vi "subDAQ_GenWaveform.vi"(7 "Waveform port selection":T2={"Dev2 DO lines"=["Dev2/port0/line3", "Dev2/port0/line5"], "Dev2 AO lines"=["Dev2/ao3", "Dev2/ao5"], "Patch AO line"="Dev1/ao0", "Dev1 AI lines"=["Dev1/ai0", "Dev1/ai8"], "Dev1 timing DO"="Dev1/port0/line1", "Camera timing DI"="Dev1/port0/line0", "Dev1 trigger source"="/Dev1/PFI0", "Dev2 trigger source"="/Dev2/PFI0"}, 8 "error in (no error)":errorcluster, 11 "Waveform info":T3={"Waveform folder"=path "C:/Users/ZouOptics/Desktop/MATLAB codes/ephys waveforms_new/Voltage triangle -100 to +50_(Baseline -30)", "Exposure time (ms)"=10.0} {"Exposure time (ms)" format="%0.5f"}) -> (0 "error out":errorcluster, 1 "Dev1 AO waveform":waveform(dbl)(graph)={"t0"=timestamp(0 s since 1904-01-01), "dt"=inf, "Y"=[]}, 2 "Lasers AO waveform":waveform(dbl)[](graph)=[{"t0"=timestamp(0 s since 1904-01-01), "dt"=inf, "Y"=[]}, {"t0"=timestamp(0 s since 1904-01-01), "dt"=inf, "Y"=[]}], 3 "Lasers DO waveform":digitalwaveform[](graph)=[{"t0"=timestamp(0 s since 1904-01-01), "dt"=inf, "Y"={"transitions"=[], "data"=[]}}, {"t0"=timestamp(0 s since 1904-01-01), "dt"=inf, "Y"={"transitions"=[], "data"=[]}}], 4 "Acquisition params":T1={"Sampling rate (Hz)"=0.0, "dt (sec)"=0.0, "total time (sec)"=0.0, "# samples"=0, "Exposure time (ms)"=1000.0, "# frames"=0} {"Exposure time (ms)" format="%0.5f"; "Sampling rate (Hz)" format="%#.3f"})   [LabVIEW 2015]
uses:
  <vilib>/Utility/file.llb/Read Delimited Spreadsheet (DBL).vi
  <vilib>/Waveform/DWDTOps.llb/DWDT Analog to Digital.vi
panel:
  in  "waveform info name":string="waveform info.txt"
  in  "waveform data name":string="waveform data.txt"
  # "Read from text file and convert columns into waveforms"
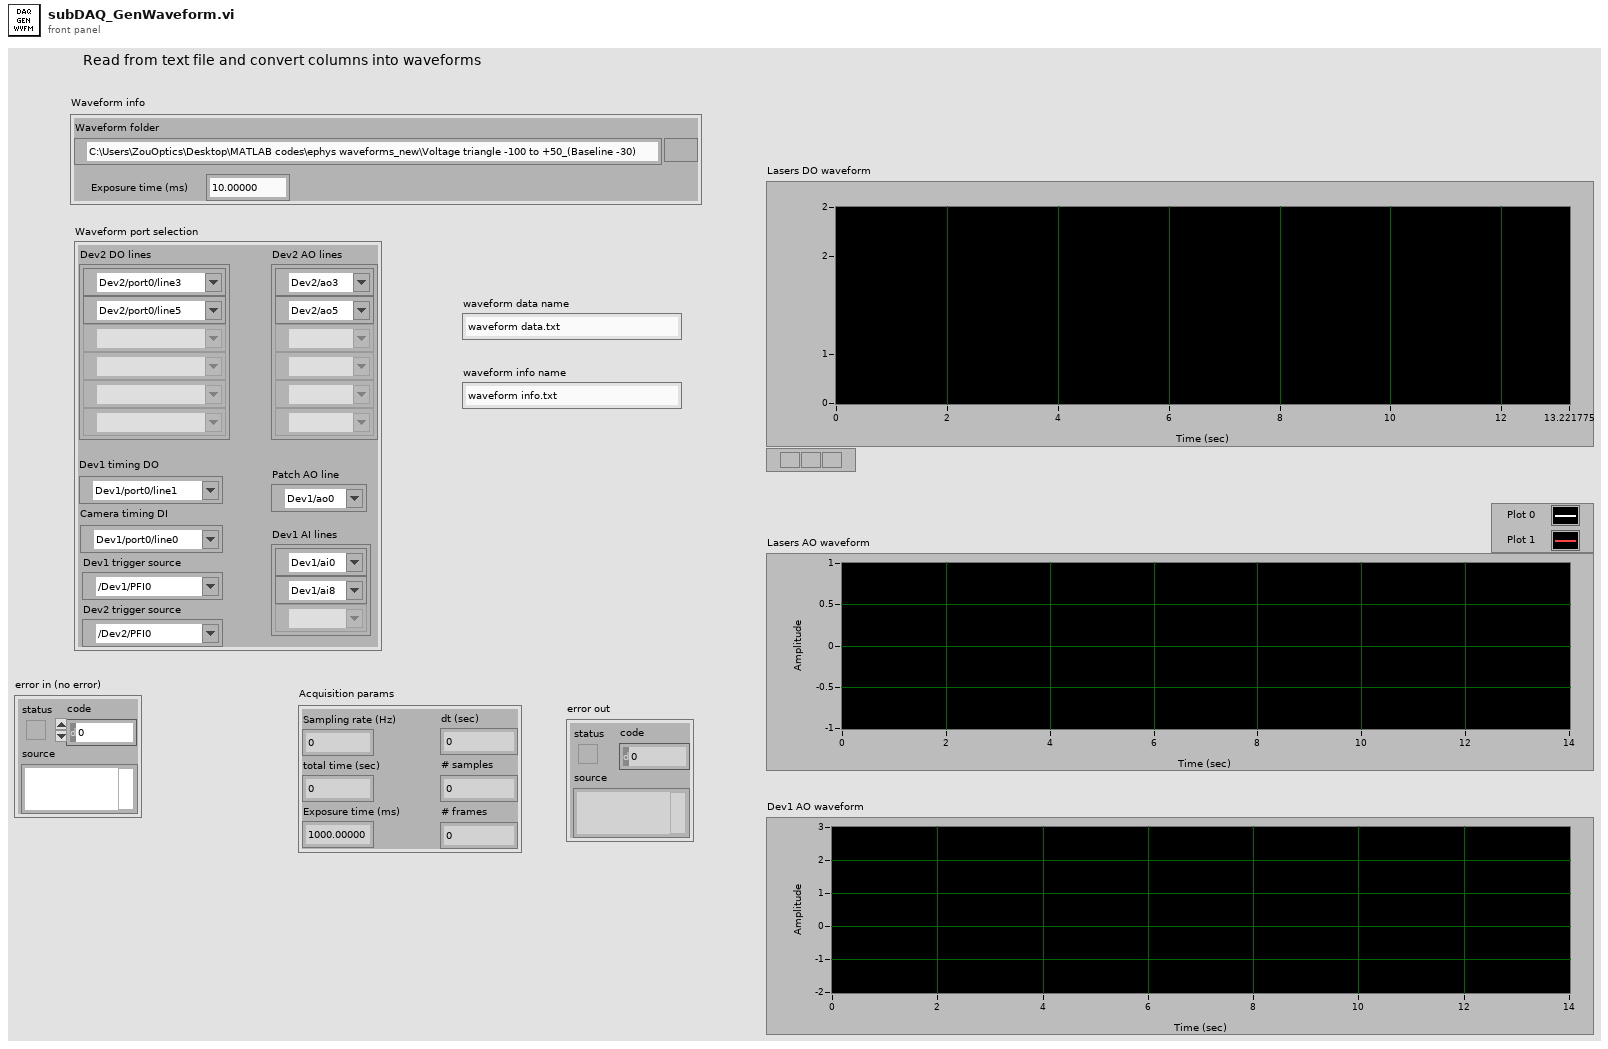
[diagram p1: front panel]
types:
  T1 = cluster{"Sampling rate (Hz)":dbl, "dt (sec)":dbl, "total time (sec)":dbl, "# samples":i32, "Exposure time (ms)":dbl, "# frames":i32}
  T2 = cluster{"Dev2 DO lines":tag[], "Dev2 AO lines":tag[], "Patch AO line":tag, "Dev1 AI lines":tag[], "Dev1 timing DO":tag, "Camera timing DI":tag, "Dev1 trigger source":tag, "Dev2 trigger source":tag}
  T3 = cluster{"Waveform folder":path, "Exposure time (ms)":dbl}
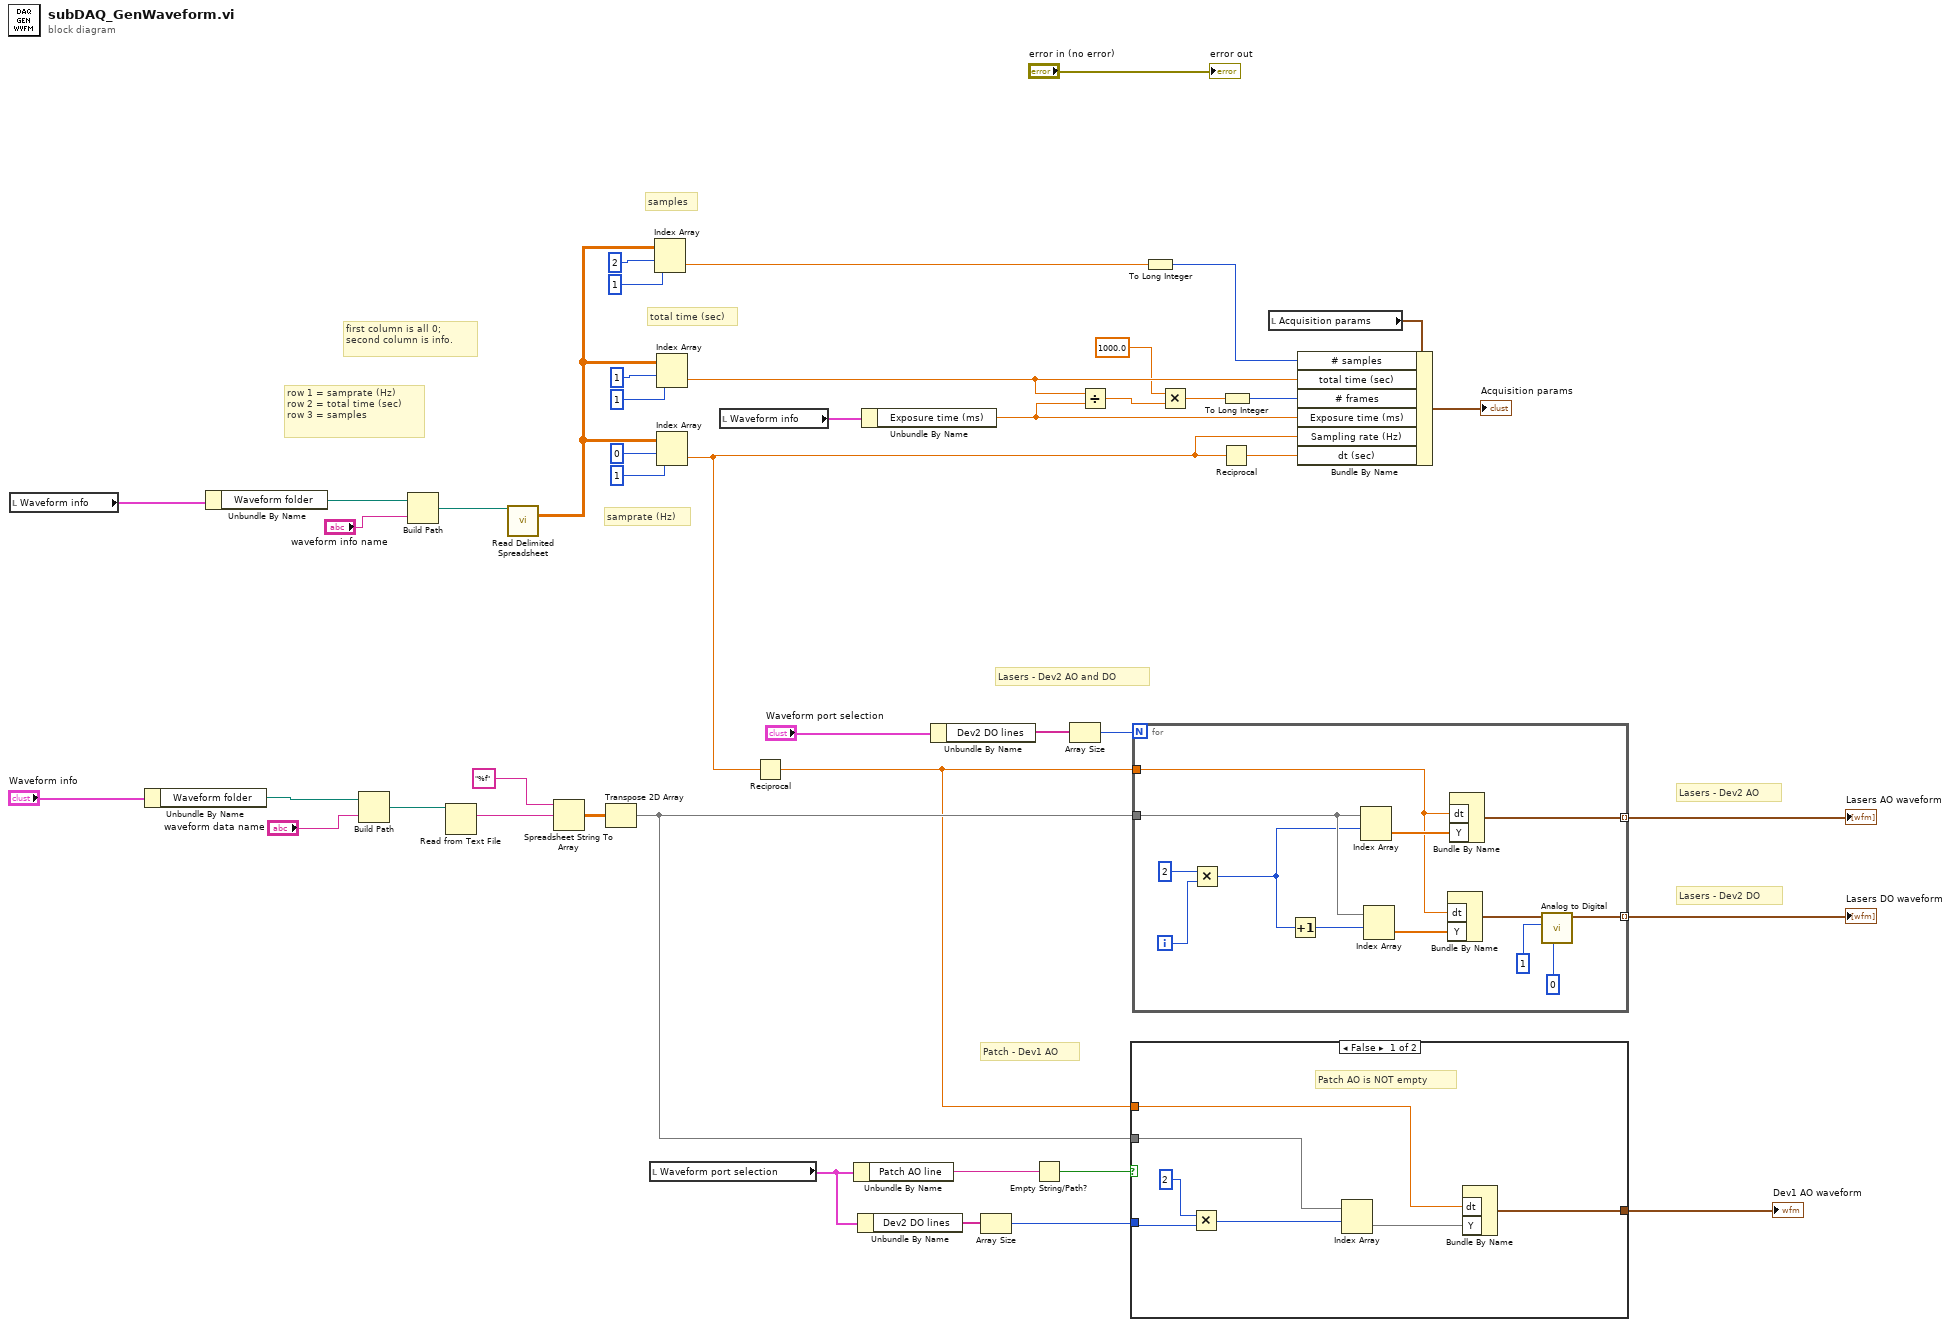
[diagram p0: block diagram]
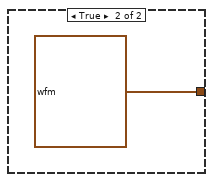
[diagram p2: hidden frame]
diagram:
  # "total time (sec)"
  # "samprate (Hz)"
  # "samples"
  # "Lasers - Dev2 AO and DO"
  # "first column is all 0;\nsecond column is info."
  # "row 1 = samprate (Hz)\nrow 2 = total time (sec)\nrow 3 = samples"
  # "Lasers - Dev2 DO"
  # "Lasers - Dev2 AO"
  # "Patch - Dev1 AO"
  n1 = local read "Waveform info"() -> (w23:T3)
  n2 = Unbundle By Name("Waveform info") -> ("Waveform folder"=w25:path)
  n3 = Unbundle By Name(w23) -> ("Waveform folder"=w21:path)
  n4 = Build Path(base path=w25, name or relative path="waveform data name") -> (appended path=w26:path)
  n5 = Build Path(base path=w21, name or relative path="waveform info name") -> (appended path=w20:path)
  n6 = Read from Text File(file (use dialog)=w26) -> (text=w45:string)  [unwired: 3 in, 3 out]
  n7 = call-poly <vilib>:"Read Delimited Spreadsheet.vi"("file path (dialog if empty)"=w20) -> ("all rows"=w11:dbl[][])  [unwired: 9 in, 5 out]
  n8 = Spreadsheet String To Array(format string="%f", spreadsheet string=w45) -> (array=w43:dbl[][])  [unwired: 2 in]
  n9 = Transpose 2D Array(2D array=w43) -> (transposed array=w27:dbl[][])
  n10 = local read "Waveform port selection"() -> (w33:T2)
  n11 = Index Array(array=w11, index (row)=2, index (col)=1 ("disabled index (col)")) -> (element=w9:dbl)
  n12 = Index Array(array=w11, index (row)=1, index (col)=1 ("disabled index (col)")) -> (element=w4:dbl)
  n13 = Index Array(array=w11, index (row)=0, index (col)=1 ("disabled index (col)")) -> (element=w7:dbl)
  n14 = local read "Waveform info"() -> (w28:T3)
  n15 = Reciprocal(x=w7) -> (1/x=w15:dbl)
  n16 = Unbundle By Name(w33) -> ("Patch AO line"=w35:tag)
  n17 = Unbundle By Name(w33) -> ("Dev2 DO lines"=w32:tag[])
  n18 = Unbundle By Name(w28) -> ("Exposure time (ms)"=w5:dbl)
  n19 = Unbundle By Name("Waveform port selection") -> ("Dev2 DO lines"=w39:tag[])
  n20 = Array Size(array=w32) -> (size(s)=w31:i32)
  n21 = Empty String/Path?(string/path=w35) -> (empty?=w34:bool)
  n22 = Array Size(array=w39) -> (size(s)=w38:i32)
  n23 = Divide(x=w4, y=w5) -> (x/y=w2:dbl)
  n24 = case shown="False" w34 {
    tunnel: w15 -> [w49 _]
    tunnel: w27 -> [w48 _]
    tunnel: w31 -> [w51 _]
    tunnel: [w47 waveform(dbl) {"t0"=timestamp(0 s since 1904-01-01), "dt"=1.0, "Y"=[]}] -> w14
    frame False {
      # "Patch AO is NOT empty"
      n25 = Multiply(x=2, y=w51) -> (x*y=w46:i32)
      n26 = Index Array(array=w48, index (row)=w46) -> (element=w52:dbl[])  [unwired: 1 in]
      n27 = Bundle By Name("dt"=w49, "Y"=w52) -> (w47:waveform(dbl))  [unwired: 1 in]
    }
    frame True {
    }
  }
  "Dev1 AO waveform" <- w14
  n28 = for {
    N: w38 -> [_]
    tunnel: w27 -> [w56]
    tunnel: [w62] -> w37 mode=indexing
    tunnel: [w57] -> w36 mode=indexing
    tunnel: w15 -> [w55]
    i -> [w66]
    n29 = Multiply(x=2, y=w66) -> (x*y=w54:i32)
    n30 = Increment(x=w54) -> (x+1=w64:i32)
    n31 = Index Array(array=w56, index (row)=w54) -> (element=w63:dbl[])  [unwired: 1 in]
    n32 = Index Array(array=w56, index (row)=w64) -> (element=w61:dbl[])  [unwired: 1 in]
    n33 = Bundle By Name("dt"=w55, "Y"=w61) -> (w58:waveform(dbl))  [unwired: 1 in]
    n34 = Bundle By Name("dt"=w55, "Y"=w63) -> (w62:waveform(dbl))  [unwired: 1 in]
    n35 = call-poly <vilib>:"Analog to Digital.vi"("data format (offset binary)"=0, "resolution (16 bit)"=1, "analog waveform"=w58) -> ("digital waveform"=w57:digitalwaveform)  [unwired: 5 in, 3 out]
  }
  "Lasers AO waveform" <- w37
  "Lasers DO waveform" <- w36
  n36 = To Long Integer(number=w9) -> (32bit integer=w10:i32)
  n37 = Multiply(x=1000.0, y=w2) -> (x*y=w1:dbl)
  n38 = Reciprocal(x=w7) -> (1/x=w8:dbl)
  n39 = To Long Integer(number=w1) -> (32bit integer=w6:i32)
  n40 = local read "Acquisition params"() -> (w29:T1)
  n41 = Bundle By Name(cluster=w29, "# samples"=w10, "total time (sec)"=w4, "# frames"=w6, "Exposure time (ms)"=w5, "Sampling rate (Hz)"=w7, "dt (sec)"=w8) -> (→"Acquisition params":T1)
  "error out" <- "error in (no error)"
